vi "Set Stage Position.vi"(3 "Position":cluster{dbl, dbl, dbl}, 4 "error in":errorcluster, 5 "VISA resource name in":refnum<visa-resource-name>) -> (1 "error out":errorcluster, 2 "VISA resource name out":refnum<visa-resource-name>)   [LabVIEW 2014]
uses:
  <vilib>/Instr/_visa.llb/VISA Configure Serial Port (Instr).vi
panel:
  out "concatenated string":string
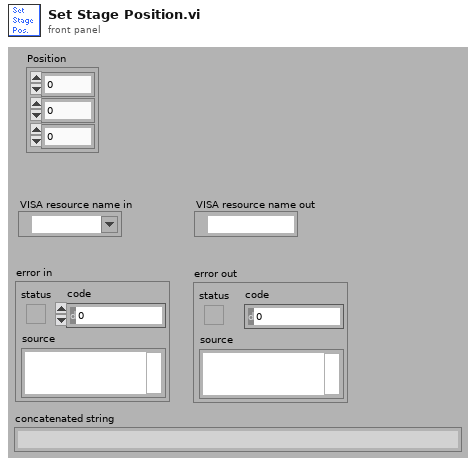
[diagram p1: front panel]
types:
  T1 = enum16{"Trackball XY", "Trackball Z", "Trackball OFF", ""}
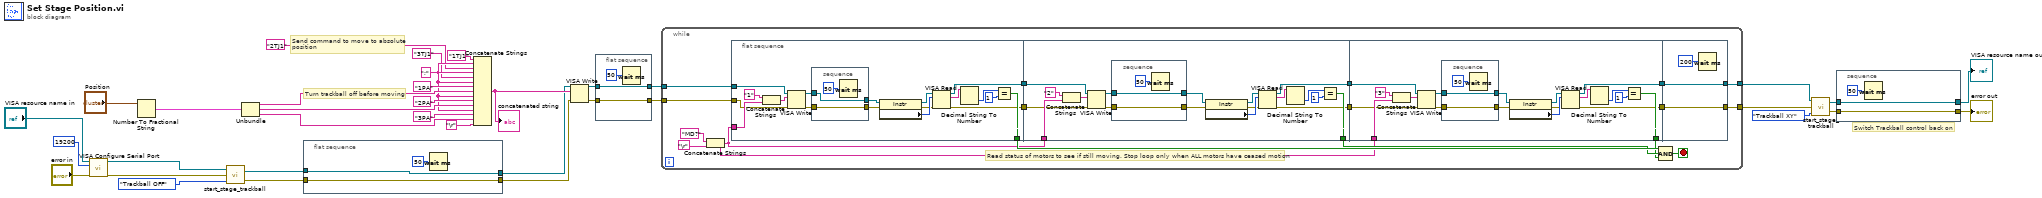
[diagram p0: block diagram]
diagram:
  w20 = ";"
  # "Switch Trackball control back on"
  # "Send command to move to absolute\nposition"
  # "Turn trackball off before moving"
  n1 = call-poly "VISA Configure Serial Port"("VISA resource name"="VISA resource name in", "baud rate (9600)"=u32 19200, "error in (no error)"="error in") -> ("VISA resource name out"=w16:refnum<visa-resource-name>, "error out"=w15:errorcluster)  [unwired: 3 in, 8 out]
  n2 = Number To Fractional String(number="Position") -> (F-format string=w29:cluster{string, string, string})  [unwired: 3 out]
  n3 = call "start_stage_trackball.vi"("Enum"=T1."Trackball OFF", "error in (no error)"=w15, "Stage Controller port"=w16) -> ("error out"=w10:errorcluster, "Stage Controller port Out"=w12:refnum<visa-resource-name>)
  n4 = Unbundle(w29) -> (w28:string, w27:string, w26:string)
  n5 = flat-sequence {
    tunnel: [w37] -> w13
    tunnel: w12 -> [w37]
    tunnel: [w36] -> w11
    tunnel: w10 -> [w36]
    frame #0 {
      n6 = Wait (ms)(milliseconds to wait=u32 50) -> ()  [unwired: 1 out]
    }
  }
  n7 = Concatenate Strings("1TJ1", w20, "2TJ1", w20, "3TJ1", w20, "1PA", w28, w20, "2PA", w27, w20, "3PA", w26, "\r") -> (w22:string)
  "concatenated string" <- w22
  n8 = VISA Write(VISA resource name=w13, write buffer=w22, error in (no error)=w11) -> (VISA resource name out=w4:refnum<visa-resource-name>, error out=w3:errorcluster)  [unwired: 1 out]
  n9 = flat-sequence {
    tunnel: [w40] -> w2
    tunnel: w4 -> [w40]
    tunnel: [w39] -> w1
    tunnel: w3 -> [w39]
    frame #0 {
      n10 = Wait (ms)(milliseconds to wait=u32 50) -> ()  [unwired: 1 out]
    }
  }
  n11 = while {
    tunnel: w2 -> [w55]
    tunnel: w1 -> [w54]
    tunnel: [w45] -> w8
    tunnel: [w44] -> w7
    stop <- w56 stop-if-true
    # "Read status of motors to see if still moving. Stop loop only when ALL motors have ceased motion"
    n12 = Concatenate Strings("MD?" ("write buffer"), "\r") -> (w49:string)
    n13 = flat-sequence {
      tunnel: w55 -> [w64]
      tunnel: w49 -> [w63]
      tunnel: w54 -> [w62]
      tunnel: [w61] -> w53
      tunnel: [w60] -> w52
      tunnel: [w59] -> w51
      tunnel: w49 -> [w85]
      tunnel: w52 -> [w84]
      tunnel: w51 -> [w83]
      tunnel: [w82] -> w50
      tunnel: [w81] -> w48
      tunnel: [w80] -> w47
      tunnel: w49 -> [w106]
      tunnel: w48 -> [w105]
      tunnel: w47 -> [w104]
      tunnel: [w103] -> w46
      tunnel: [w102] -> w43
      tunnel: [w101] -> w42
      tunnel: [w123] -> w44
      tunnel: [w124] -> w45
      tunnel: w43 -> [w124]
      tunnel: w42 -> [w123]
      frame #0 {
        n14 = Concatenate Strings("1" ("string"), w63) -> (w76:string)
        n15 = VISA Write(VISA resource name=w64, write buffer=w76, error in (no error)=w62) -> (VISA resource name out=w73:refnum<visa-resource-name>, error out=w72:errorcluster)  [unwired: 1 out]
        n16 = stacked-sequence {
          tunnel: [w79] -> w71
          tunnel: w73 -> [w79]
          tunnel: w72 -> [w78]
          tunnel: [w78] -> w67
          frame #0 {
            n17 = Wait (ms)(milliseconds to wait=50) -> ()  [unwired: 1 out]
          }
        }
        n18 = property class="Instr"(reference=w71, error in=w67) -> (reference out=w70:refnum<visa-resource-name>, error out=w68:errorcluster, "Serial Settings:Number of Bytes at Serial Port"=w69:u32)
        n19 = VISA Read(VISA resource name=w70, byte count=w69, error in (no error)=w68) -> (VISA resource name out=w60:refnum<visa-resource-name>, read buffer=w74:string, error out=w59:errorcluster)  [unwired: 1 out]
        n20 = Decimal String To Number(string=w74) -> (number=w66:i32)  [unwired: 3 out]
        n21 = Equal?(x=w66, y=1) -> (x = y?=w61:bool)
      }
      frame #1 {
        n22 = Concatenate Strings("2" ("string"), w85) -> (w97:string)
        n23 = VISA Write(VISA resource name=w84, write buffer=w97, error in (no error)=w83) -> (VISA resource name out=w94:refnum<visa-resource-name>, error out=w93:errorcluster)  [unwired: 1 out]
        n24 = stacked-sequence {
          tunnel: [w100] -> w92
          tunnel: w94 -> [w100]
          tunnel: w93 -> [w99]
          tunnel: [w99] -> w88
          frame #0 {
            n25 = Wait (ms)(milliseconds to wait=50) -> ()  [unwired: 1 out]
          }
        }
        n26 = property class="Instr"(reference=w92, error in=w88) -> (reference out=w91:refnum<visa-resource-name>, error out=w89:errorcluster, "Serial Settings:Number of Bytes at Serial Port"=w90:u32)
        n27 = VISA Read(VISA resource name=w91, byte count=w90, error in (no error)=w89) -> (VISA resource name out=w81:refnum<visa-resource-name>, read buffer=w95:string, error out=w80:errorcluster)  [unwired: 1 out]
        n28 = Decimal String To Number(string=w95) -> (number=w87:i32)  [unwired: 3 out]
        n29 = Equal?(x=w87, y=1) -> (x = y?=w82:bool)
      }
      frame #2 {
        n30 = Concatenate Strings("3" ("string"), w106) -> (w118:string)
        n31 = VISA Write(VISA resource name=w105, write buffer=w118, error in (no error)=w104) -> (VISA resource name out=w115:refnum<visa-resource-name>, error out=w114:errorcluster)  [unwired: 1 out]
        n32 = stacked-sequence {
          tunnel: [w121] -> w113
          tunnel: w115 -> [w121]
          tunnel: w114 -> [w120]
          tunnel: [w120] -> w109
          frame #0 {
            n33 = Wait (ms)(milliseconds to wait=50) -> ()  [unwired: 1 out]
          }
        }
        n34 = property class="Instr"(reference=w113, error in=w109) -> (reference out=w112:refnum<visa-resource-name>, error out=w110:errorcluster, "Serial Settings:Number of Bytes at Serial Port"=w111:u32)
        n35 = VISA Read(VISA resource name=w112, byte count=w111, error in (no error)=w110) -> (VISA resource name out=w102:refnum<visa-resource-name>, read buffer=w116:string, error out=w101:errorcluster)  [unwired: 1 out]
        n36 = Decimal String To Number(string=w116) -> (number=w108:i32)  [unwired: 3 out]
        n37 = Equal?(x=w108, y=1) -> (x = y?=w103:bool)
      }
      frame #3 {
        n38 = Wait (ms)(milliseconds to wait=u32 200) -> ()  [unwired: 1 out]
      }
    }
    n39 = Compound Arithmetic op=AND(w53, w50, w46) -> (w56:bool)
  }
  n40 = call "start_stage_trackball.vi"("Enum"=T1."Trackball XY", "error in (no error)"=w7, "Stage Controller port"=w8) -> ("error out"=w5:errorcluster, "Stage Controller port Out"=w6:refnum<visa-resource-name>)
  n41 = stacked-sequence {
    tunnel: [w127] -> w32
    tunnel: w6 -> [w127]
    tunnel: w5 -> [w126]
    tunnel: [w126] -> w31
    frame #0 {
      n42 = Wait (ms)(milliseconds to wait=50) -> ()  [unwired: 1 out]
    }
  }
  "VISA resource name out" <- w32
  "error out" <- w31
